vi "拷贝到预备区.vi"(9 "Coords":T1, 11 "CtlRef":refnum<vi>) -> (1 "预备区功率":string, 3 "衰减/偏置":u32[](array[numeric]))   [LabVIEW 2015]
uses:
  <vilib>/Utility/miscctls.llb/LVPoint32TypeDef.ctl
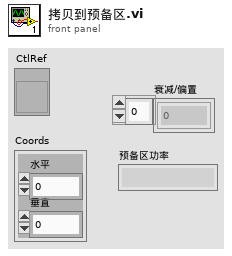
[diagram p1: front panel]
types:
  T1 = typedef "LVPoint32TypeDef.ctl" = cluster{"Horizontal":i32, "Vertical":i32}
  T2 = typedef "LVRowAndColumnTypeDef.ctl" = cluster{"Row":i32, "Column":i32}
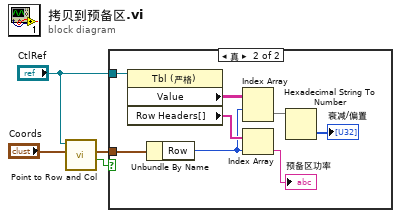
[diagram p0: block diagram]
diagram:
  n1 = call "Point to Row and Col.vi"("点"="Coords", "Table Ref In"="CtlRef") -> ("边界内？"=w2:bool, "单元格位置"=w3:T2)  [unwired: 6 in, 2 out]
  n2 = case shown="真" w2 {
    tunnel: w3 -> [_ w12]
    tunnel: "CtlRef" -> [_ w11]
    frame False {
    }
    frame True {
      n3 = property class="Tbl (严格)"(reference=w11) -> ("Value"=w9:string[][], "Row Headers[]"=w10:string[])  [unwired: 1 in, 2 out]
      n4 = Unbundle By Name(w12) -> ("Row"=w8:i32)
      n5 = Index Array(array=w9, index (row)=w8) -> (element=w6:string[])  [unwired: 1 in]
      n6 = Index Array(array=w10, index=w8) -> (element=→"预备区功率":string)
      n7 = Hexadecimal String To Number(string=w6) -> (number=→"衰减/偏置":u32[])  [unwired: 2 in, 1 out]
    }
  }
